vi "VTI_Set_Monitor_Values.vi"(4 "VTI Status":T1={"Temperatur (K)"=70.6986, "Heater (%)"=0.0017142857142857142, "NV (%)"=0.0, "Heater Manual"=TRUE, "NV Manual"=TRUE, "Pressure"=1.0208606, "Valid?"=FALSE, "Heater (%) Display"=0.0, "NV (%) Display"=0.0, "Sample 2"=70.6986, "Sample 3"=70.6986, "Auto PID"=TRUE, "Sweep-Status"=TRUE, "Setpoint-Sweep"=70.6986} {"Heater (%)" scale=0.0..100.0; "NV (%)" scale=0.0..100.0}, 5 "System Monitor Variables (in)":T2) -> (1 "System Monitor Variables (out)":T2)   [LabVIEW 2016]
uses:
  Global/Global Variables/System Monitor Cluster.ctl
  S16/VTI-status.ctl
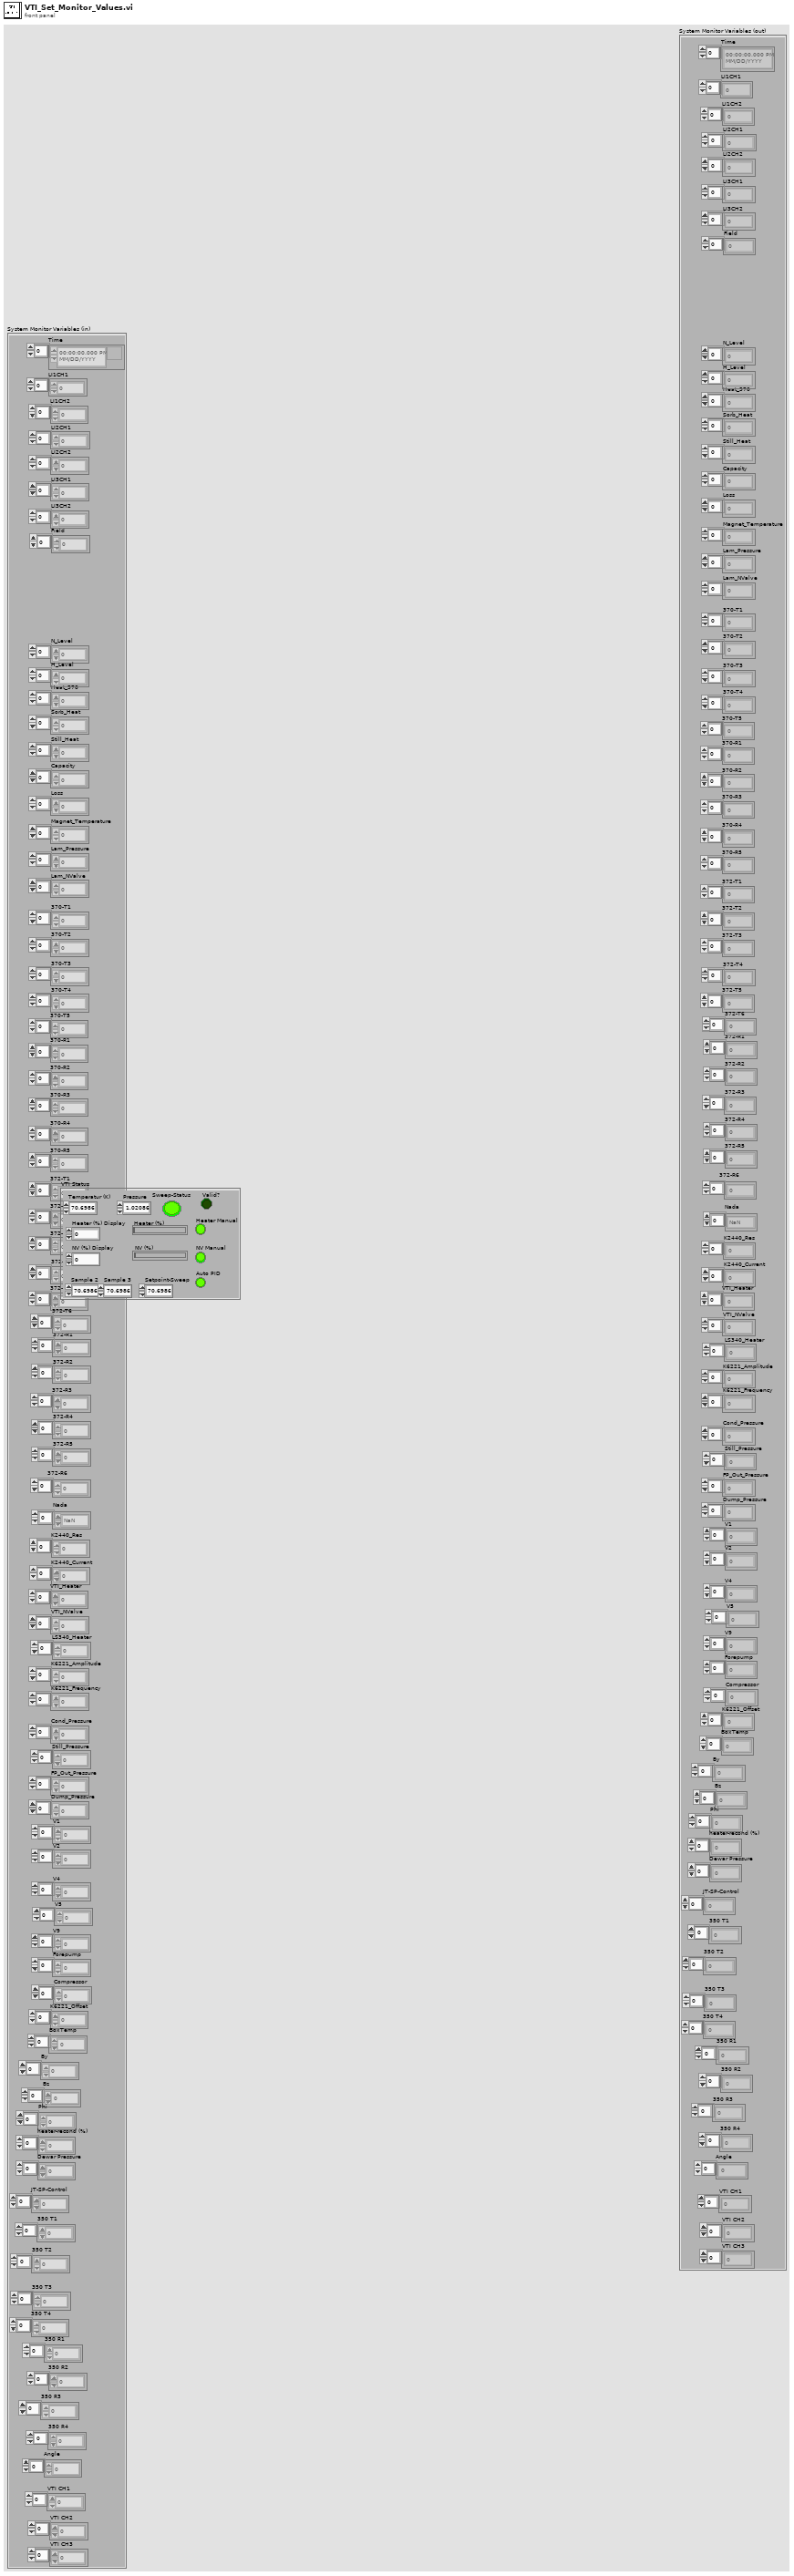
[diagram p1: front panel]
types:
  T1 = typedef "VTI-status.ctl" = cluster{"Temperatur (K)":dbl, "Heater (%)":dbl, "NV (%)":dbl, "Heater Manual":bool, "NV Manual":bool, "Pressure":dbl, "Valid?":bool, "Heater (%) Display":dbl, "NV (%) Display":dbl, "Sample 2":dbl, "Sample 3":dbl, "Auto PID":bool, "Sweep-Status":bool, "Setpoint-Sweep":dbl}
  T2 = typedef "System Monitor Cluster.ctl" = cluster{"Time":timestamp[], "LI1CH1":dbl[], "LI1CH2":dbl[], "LI2CH1":dbl[], "LI2CH2":dbl[], "LI3CH1":dbl[], "LI3CH2":dbl[], "Field":dbl[], "N_Level":dbl[], "H_Level":dbl[], "Heat_370":dbl[], "Sorb_Heat":dbl[], "Still_Heat":dbl[], "Capacity":dbl[], "Loss":dbl[], "Magnet_Temperature":dbl[], "Lam_Pressure":dbl[], "Lam_NValve":dbl[], "370-T1":dbl[], "370-T2":dbl[], "370-T3":dbl[], "370-T4":dbl[], "370-T5":dbl[], "370-R1":dbl[], "370-R2":dbl[], "370-R3":dbl[], "370-R4":dbl[], "370-R5":dbl[], "372-T1":dbl[], "372-T2":dbl[], "372-T3":dbl[], "372-T4":dbl[], "372-T5":dbl[], "372-T6":dbl[], "372-R1":dbl[], "372-R2":dbl[], "372-R3":dbl[], "372-R4":dbl[], "372-R5":dbl[], "372-R6":dbl[], "Nada":dbl[], "K2440_Res":dbl[], "K2440_Current":dbl[], "VTI_Heater":dbl[], "VTI_NValve":dbl[], "LS340_Heater":dbl[], "K6221_Amplitude":dbl[], "K6221_Frequency":dbl[], "Cond_Pressure":dbl[], "Still_Pressure":dbl[], "FP_Out_Pressure":dbl[], "Dump_Pressure":dbl[], "V1":dbl[], "V2":dbl[], "V4":dbl[], "V5":dbl[], "V9":dbl[], "Forepump":dbl[], "Compressor":dbl[], "K6221_Offset":dbl[], "BoxTemp":dbl[], "By":dbl[], "Bz":dbl[], "Phi":dbl[], "heater-recond (%)":dbl[], "Dewar Pressure ":dbl[], "JT-SP-Control":dbl[], "350 T1":dbl[], "350 T2":dbl[], "350 T3":dbl[], "350 T4":dbl[], "350 R1":dbl[], "350 R2":dbl[], "350 R3":dbl[], "350 R4":dbl[], "Angle":dbl[], "VTI CH1":dbl[], "VTI CH2":dbl[], "VTI CH3":dbl[]}
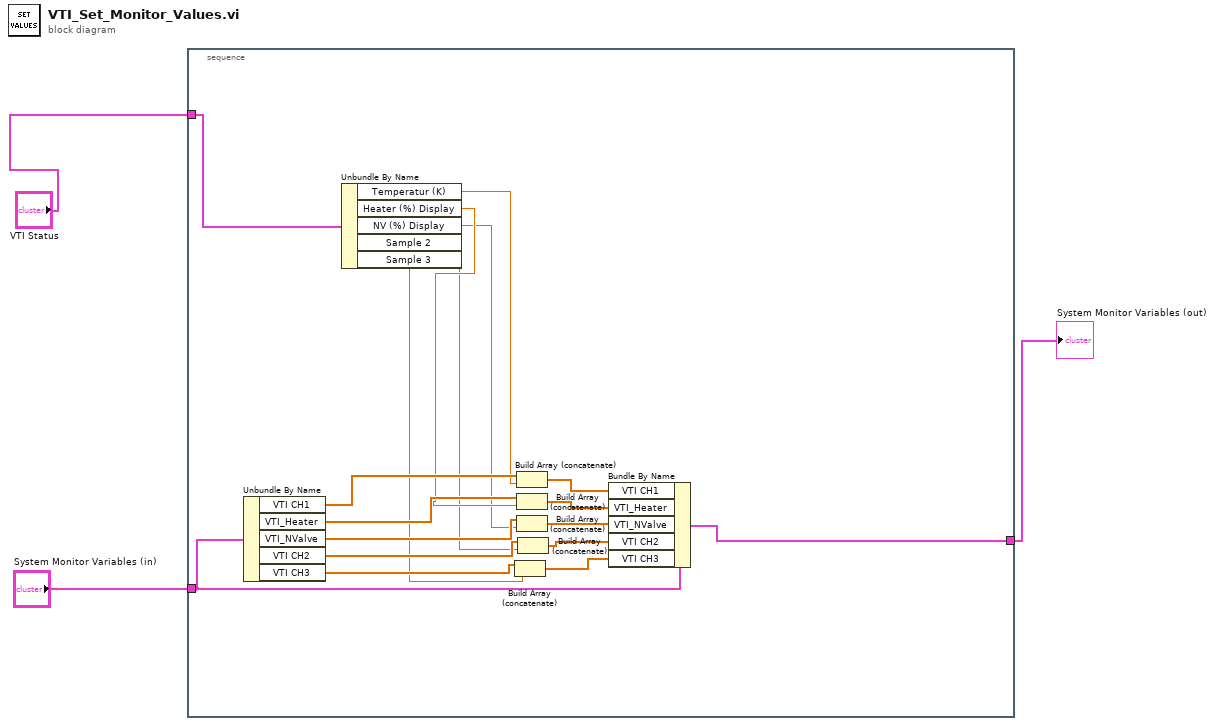
[diagram p0: block diagram]
diagram:
  n1 = stacked-sequence {
    tunnel: "System Monitor Variables (in)" -> [w11]
    tunnel: [w15] -> w2
    tunnel: "VTI Status" -> [w10]
    frame #0 {
      n2 = Unbundle By Name(w11) -> ("VTI CH1"=w21:dbl[], "VTI_Heater"=w20:dbl[], "VTI_NValve"=w19:dbl[], "VTI CH2"=w9:dbl[], "VTI CH3"=w8:dbl[])
      n3 = Unbundle By Name(w10) -> ("Temperatur (K)"=w18:dbl, "Heater (%) Display"=w17:dbl, "NV (%) Display"=w16:dbl, "Sample 2"=w4:dbl, "Sample 3"=w5:dbl)
      n4 = Build Array (concatenate)(w8, w5) -> (w6:dbl[])
      n5 = Build Array (concatenate)(w21, w18) -> (w14:dbl[])
      n6 = Build Array (concatenate)(w20, w17) -> (w13:dbl[])
      n7 = Build Array (concatenate)(w19, w16) -> (w12:dbl[])
      n8 = Build Array (concatenate)(w9, w4) -> (w7:dbl[])
      n9 = Bundle By Name(cluster=w11, "VTI CH1"=w14, "VTI_Heater"=w13, "VTI_NValve"=w12, "VTI CH2"=w7, "VTI CH3"=w6) -> (w15:T2)
    }
  }
  "System Monitor Variables (out)" <- w2
